vi "remote.Get Property DataType.vi"(0 "SLSC Remote in":refnum<class "SLSC Interface.lvclass">, 5 "property":refnum<k21>, 11 "error in (no error)":errorcluster) -> (4 "SLSC Remote out":refnum<class "SLSC Interface.lvclass">, 6 "property out":refnum<k21>, 10 "Prop.DataType":i32(ring) items=["None", "Bool", "DBL", "I32", "I64", "String", "U32", "U64", "1D Bool", "1D DBL", "1D I32", "1D I64", "1D String", "1D U32", "1D U64"], 15 "error out":errorcluster)   [LabVIEW 2016, in "SLSC Interfaces.lvlib" / "SLSC Interface.lvclass"]
uses:
  SLSC Interface Class/SLSC Interface.lvclass
  <vilib>/NI/NI JSONRPC Server Framework/Classes/Server/JSONRPC Server.lvclass
  <vilib>/httpClient/LabVIEWHTTPClient.lvlib
  <vilib>/NI/JSON Support for LabVIEW/JSON Data Classes/JSON Object/JSON Object.lvclass
  <vilib>/httpClient/POSTBuffer.vi
  <vilib>/NI/JSON Support for LabVIEW/JSON Data Classes/JSON Object/Get Value (String Value).vi
  <vilib>/NI/JSON Support for LabVIEW/JSON Data Classes/JSON Helper/JSON Helper.lvclass
  <vilib>/NI/JSON Support for LabVIEW/JSON Data Classes/JSON Object/New JSON Object (Multi String).vi
  <vilib>/NI/NI JSONRPC Server Framework/Classes/Server/Format Client Request (Auto-Increment).vi
  <vilib>/NI/NI JSONRPC Server Framework/Classes/Server/Parse Response (Object).vi
  C:/Program Files (x86)/National Instruments/LabVIEW 2016/vi.lib/NI/JSON Support for LabVIEW/JSON Data Classes/JSON Structured Type/JSON Structure.lvclass
  C:/Program Files (x86)/National Instruments/LabVIEW 2016/vi.lib/NI/JSON Support for LabVIEW/JSON Data Classes/JSON Datatype/JSON Null.lvclass
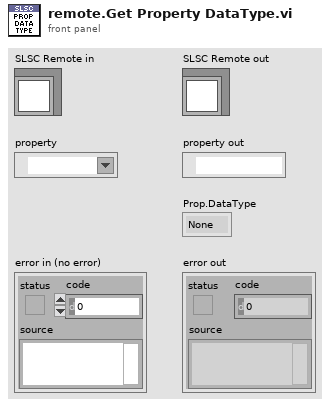
[diagram p1: front panel]
types:
  T1 = typedef "LabVIEWHTTPClient.lvlib/ClientHandle.ctl" = refnum<k1>
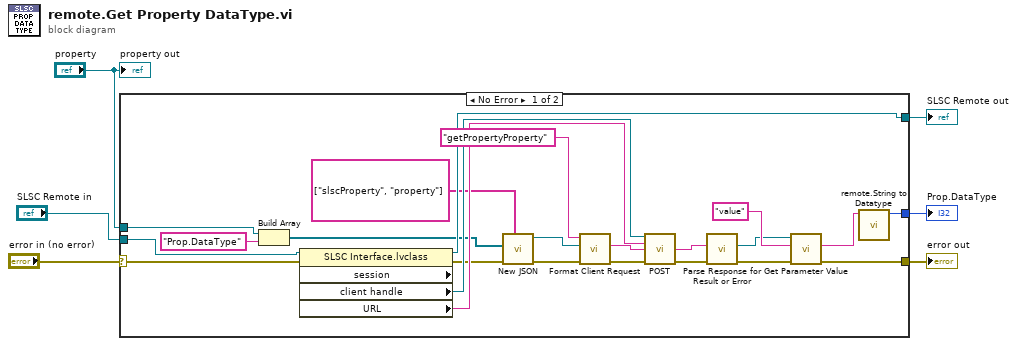
[diagram p0: block diagram]
diagram:
  n1 = case shown="No Error" "error in (no error)" {
    selector: "error in (no error)" -> [w27 w30]
    tunnel: "SLSC Remote in" -> [w29 w31]
    tunnel: [w28 w31] -> w2
    tunnel: [w19 w30] -> w4
    tunnel: "property" -> [w13 _]
    tunnel: [w17 _] -> w1
    frame No Error {
      n2 = Build Array(w13, "Prop.DataType" ("String")) -> (w11:refnum<k21>[])
      n3 = property class="SLSC Interface.lvclass" props=["session", "client handle", "URL"](reference=w29, error in=w27) -> (reference out=w28:refnum<class "SLSC Interface.lvclass">, error out=w10:errorcluster, "client handle"=w24:T1, "URL"=w23:string)  [unwired: 1 out]
      n4 = call-poly <vilib>:"New JSON.vi"("keys"=string[] ["slscProperty", "property"], "error in (no error)"=w10, "values"=w11) -> ("error out"=w9:errorcluster, "JSON Object out"=w8:refnum<class "JSON Object.lvclass">)  [unwired: 7 in]
      n5 = call-poly <vilib>:"Format Client Request.vi"("error in (no error)"=w9, "JSON in"=w8, "method"="getPropertyProperty") -> ("error out"=w22:errorcluster, "Request String"=w25:string)  [unwired: 7 in]
      n6 = call-poly <vilib>:"POST.vi"("client handle"=w24, "url"=w23, "buffer"=w25, "error in (no error)"=w22) -> ("body"=w21:string, "error out"=w20:errorcluster)  [unwired: 8 in, 2 out]
      n7 = call-poly <vilib>:"Parse Response for Result or Error.vi"("error in"=w20, "Response String In"=w21) -> ("error out"=w15:errorcluster, "JSON Array"=w7:refnum<class "JSON Object.lvclass">)  [unwired: 7 in, 1 out]
      n8 = call-poly <vilib>:"Get Parameter Value.vi"("error in (no error)"=w15, "key"="value" ("Parameter Name"), "JSON Object in"=w7) -> ("error out"=w19:errorcluster, "value"=w16:string)  [unwired: 7 in]
      n9 = call "remote.String to Datatype.vi"("String Value"=w16) -> ("Prop.DataType"=w17:i32)  [unwired: 10 in]
    }
    frame Error {
    }
  }
  "error out" <- w4
  "SLSC Remote out" <- w2
  "Prop.DataType" <- w1
  "property out" <- "property"
